vi "HumanNetwork.vi"   [LabVIEW 2020]
uses:
  <vilib>/Rock Robotics/Network Tables/NT Read Boolean.vi
  HumanGlobal.vi
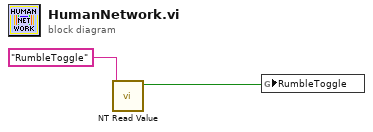
[diagram p0: block diagram]
diagram:
  n1 = call-poly <vilib>:"NT Read Value.vi"("Name"="RumbleToggle") -> ("Boolean"=w1:bool)  [unwired: 9 in, 1 out]
  n2 = global write "HumanGlobal.vi" "RumbleToggle"(w1) -> ()
